vi "MCLScanAPD.vi"(0 "Image In":T1(plugin-control)=refnum caption="APD 1 (Cy3)", 1 "APD Cts":dbl[](array[numeric]), 2 "Scan steps (MCL)":u64=40 caption="Scan steps (x)", 3 "Scan lines (y)":u64=20, 4 "N APD Samp/step":i32=3, 5 "NewScan?":bool) -> (14 "Image Out":T1(plugin-control) caption="APD 1 (Cy3)")   [LabVIEW 2013]
uses:
  <vilib>/Analysis/baseanly.llb/Mean (DBL).vi
  <vilib>/vision/NI_Vision_Development_Module.lvlib
  <vilib>/Analysis/NI_AALBase.lvlib
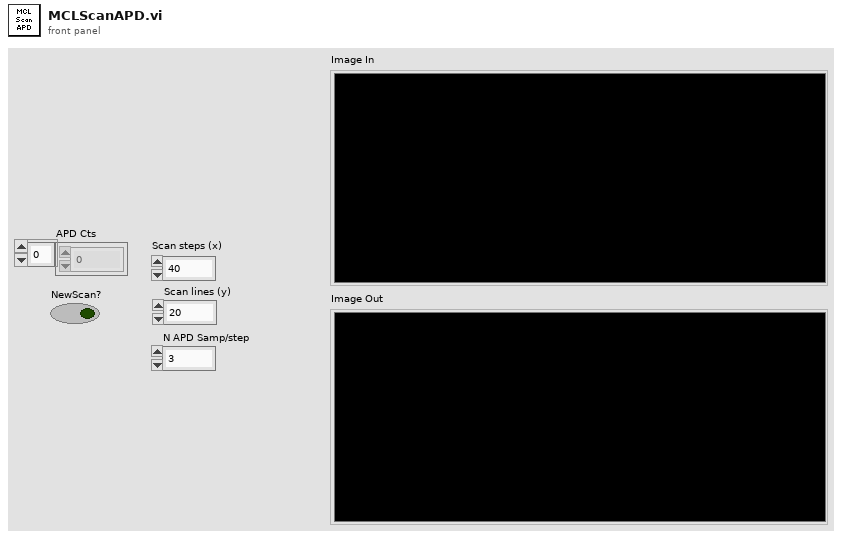
[diagram p1: front panel]
types:
  T1 = typedef "IMAQ Image.ctl" = refnum<image>
  T2 = cluster{"Origin Pixel":cluster{"X":sgl, "Y":sgl}, "Angle Relative to Horizontal (deg)":sgl, "Axis Reference":u32}
  T3 = typedef "Simple Grid Descriptor" = cluster{"X Step":sgl, "Y Step":sgl, "Unit":T4}
  T4 = typedef "Image Unit" = enum32{"Undefined", "Angström", "Micrometer", "Millimeter", "Centimeter", "Meter", "Kilometer", "Microinch", "Inch", "Feet", "Nautical miles", "Standard miles", "Steps"}
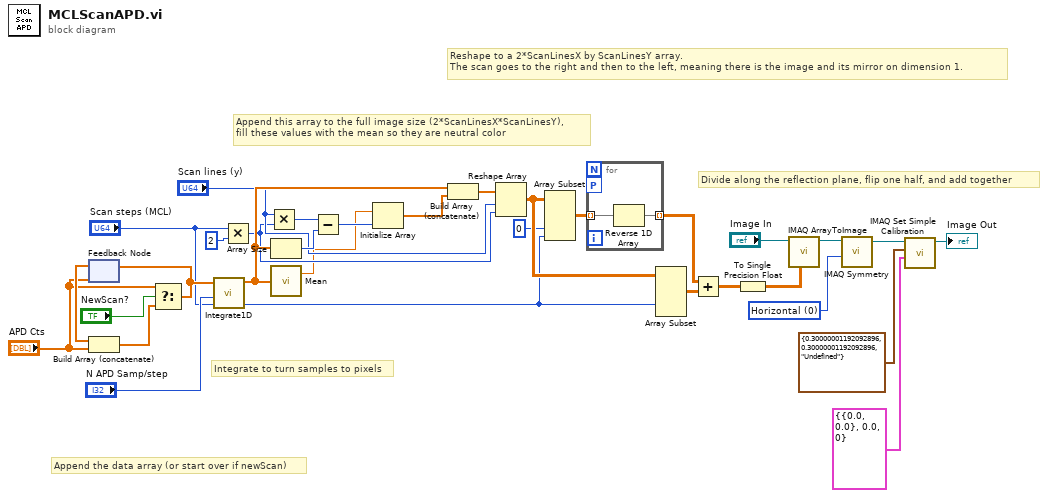
[diagram p0: block diagram]
diagram:
  w24 = u32 0 items=["Horizontal", "Vertical", "Central", "1st Diagonal", "2nd Diagonal"] ("Type of Symmetry")
  # "Divide along the reflection plane, flip one half, and add together"
  # "Reshape to a 2*ScanLinesX by ScanLinesY array.\nThe scan goes to the right and then to the left, meaning there is the image and its mirror on dimension 1."
  # "Append this array to the full image size (2*ScanLinesX*ScanLinesY),\nfill these values with the mean so they are neutral color"
  # "Integrate to turn samples to pixels"
  # "Append the data array (or start over if newScan)"
  n1 = feedback #1("APD Cts") -> (w11:dbl[])
  n2 = Build Array (concatenate)(w11, "APD Cts") -> (w17:dbl[])
  n3 = Select(t="APD Cts", s="NewScan?", f=w17) -> (s? t:f=w15:dbl[])
  n4 = feedback-in #1(w15) -> ()
  n5 = call "Integrate1D.vi"("Avg N"="N APD Samp/step", "Array In"=w15) -> ("Array Out"=w16:dbl[])  [unwired: 9 in]
  n6 = Multiply(x="Scan steps (MCL)", y=u64 2) -> (x*y=w3:u64)
  n7 = Multiply(x="Scan lines (y)", y=w3) -> (x*y=w12:u64)
  n8 = Array Size(array=w16) -> (size(s)=w14:i32)
  n9 = call-poly <vilib>:"Mean.vi"("X"=w16) -> ("mean"=w2:dbl)  [unwired: 1 out]
  n10 = Subtract(x=w12, y=w14) -> (x-y=w30:u64)
  n11 = Initialize Array(w2, w30) -> (w1:dbl[])
  n12 = Build Array (concatenate)(w16, w1) -> (w13:dbl[])
  n13 = Reshape Array(w13, "Scan lines (y)", w3) -> (w19:dbl[][])
  n14 = Array Subset(array=w19, index (col)=0 ("index"), length (col)="Scan steps (MCL)") -> (w20:dbl[][])  [unwired: 2 in]
  n15 = for {
    tunnel: w20 -> [w33] mode=indexing
    tunnel: [w32] -> w21 mode=indexing
    workers-P: _ -> [_]
    n16 = Reverse 1D Array(array=w33) -> (reversed array=w32:dbl[])
  }
  n17 = Array Subset(array=w19, index (col)="Scan steps (MCL)") -> (w22:dbl[][])  [unwired: 3 in]
  n18 = Add(x=w21, y=w22) -> (x+y=w25:dbl[][])
  n19 = To Single Precision Float(number=w25) -> (single precision float=w26:sgl[][])
  n20 = call "IMAQ ArrayToImage"("Image Pixels (Float)"=w26, "Image"="Image In") -> ("Image Out"=w23:T1)  [unwired: 8 in, 1 out]
  n21 = call "IMAQ Symmetry"("Type of Symmetry"=w24, "Image Src"=w23) -> ("Image Dst Out"=w28:T1)  [unwired: 3 in, 1 out]
  n22 = call "IMAQ Set Simple Calibration"("Calibration Axis Info"=T2 {"Origin Pixel"={"X"=0.0, "Y"=0.0}, "Angle Relative to Horizontal (deg)"=0.0, "Axis Reference"=0}, "Grid Descriptor"=T3 {"X Step"=0.3, "Y Step"=0.3, "Unit"=enum."Undefined"}, "Image"=w28) -> ("Calibrated Image"=→"Image Out":T1)  [unwired: 7 in, 1 out]
